vi "Transmission.vi"() -> ()   [LabVIEW 2016, in "beamline sections.lvlib" / "transmission.lvlib"]
uses:
  Transmission/transmission.lvlib
  save load/saveloadprev.ctl
  controls/Faraday cup states.ctl
  <vilib>/Instr/_visa.llb/VISA Open Access Mode.ctl
  low energy end/Low energy end/Low energy end llb.lvlib
  High energy end/High energy llb.lvlib
  save load/SaveLoad.lvlib
panel:
  in  "Tab Control":T1(tab)
  in  "ExB Electric":dbl(slide) min=0.0 max=200.0 scale=0.0..60.0
  out "Trans Steerer Y Read":dbl format="%#.3g"
  out "Trans Steerer X Read":dbl format="%#.3g"
  in  "Transmission Y steerer":dbl(slide) min=-10.0 max=10.0 scale=-10.0..10.0
  in  "Transmission Quad A":dbl(slide) min=0.0 max=200.0 scale=0.0..120.0
  out "Switch magnet":bool=TRUE
  in  "Transmission X steerer":dbl(slide) min=-10.0 max=10.0 scale=-10.0..10.0
  out "Transmission Steerer":bool
  out "Transmission quad Range":bool
  in  "Transmission Quad B":dbl(slide) min=0.0 max=200.0 scale=0.0..120.0
  in  "stop":bool
  out "ExB":bool
  out "ExB Voltage Read-":dbl format="%#.3g"
  in  "ExB Magnet":dbl(slide) scale=0.0..10.0
  out "ExB Voltage Read +":dbl format="%#.3g"
  in  "Switch magnet set":dbl(slide) min=0.0 max=1.6 scale=0.0..1.0
  out "Switch magnet readback":dbl(graph)
  out "Quad A I read":string
  out "Quad A V read":string
  out "Quad B I read":string
  out "Quad B V read":string
  in  "Preview-Save-Load":T2
  out "ExB Magnet read":dbl
  out "R30 Switch magnet FC status":T3
  out "Switch Mag PS output setting":dbl
  in  "Trans temp file":path=path "D:/Main Tune Parameters/Temp Configs/Transmission.txt"
  in  "Quad A - VISA GPIB Resource":refnum<visa-resource-name>="GPIB2::8::INSTR"
  in  "Quad B - VISA GPIB Resource":refnum<visa-resource-name>="GPIB2::12::INSTR"
  out "ExB +READ I":dbl
  out "ExB - I":dbl
  out "Trans steer +X I":dbl
  out "Trans steer -X  I":dbl
  out "Trans steer +Y I":dbl
  out "Trans steer -Y I":dbl
  out "Trans steer +X":dbl
  out "Trans steer -X":dbl
  out "Trans steer +X Set":dbl
  out "Trans steer -X Set":dbl
  out "Trans steer +Y":dbl
  out "Trans steer -Y":dbl
  out "Trans steer +Y Set":dbl
  out "Trans steer -Y Set":dbl
  out "Quad B error":errorcluster
  out "Quad A error":errorcluster
  out "SaveLoad error":errorcluster
  out "SV error - event loop":errorcluster
  out "SV error - while loop":errorcluster
  out "Trans-RT Error":errorcluster
  out "Trans-FPGA Error":errorcluster
  # "Transmission"
  # "Quad A initially set to GPIB2::8\nQuad B initially set to GPIB2::12"
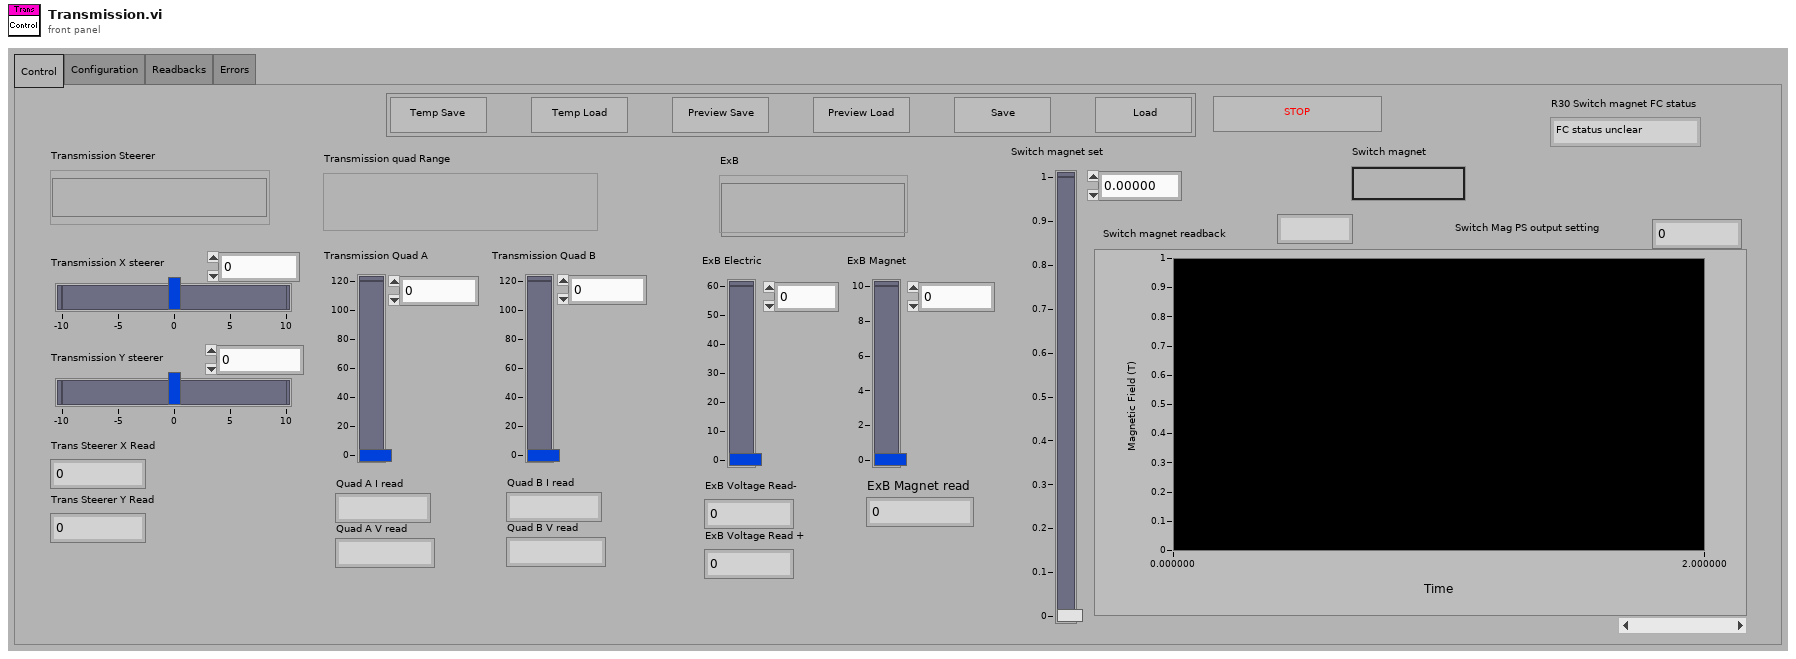
[diagram p1: front panel]
types:
  T1 = enum32{"Control", "Configuration", "Readbacks", "Errors"}
  T2 = typedef "saveloadprev.ctl" = cluster{"Temp Save":bool, "Temp Load":bool, "Save":bool, "Load":bool, "Preview Save":bool, "Preview Load":bool}
  T3 = typedef "Faraday cup states.ctl" = enum16{"FC status unclear", "FC in", "FC out"}
  T4 = typedef "VISA Open Access Mode.ctl" = u32
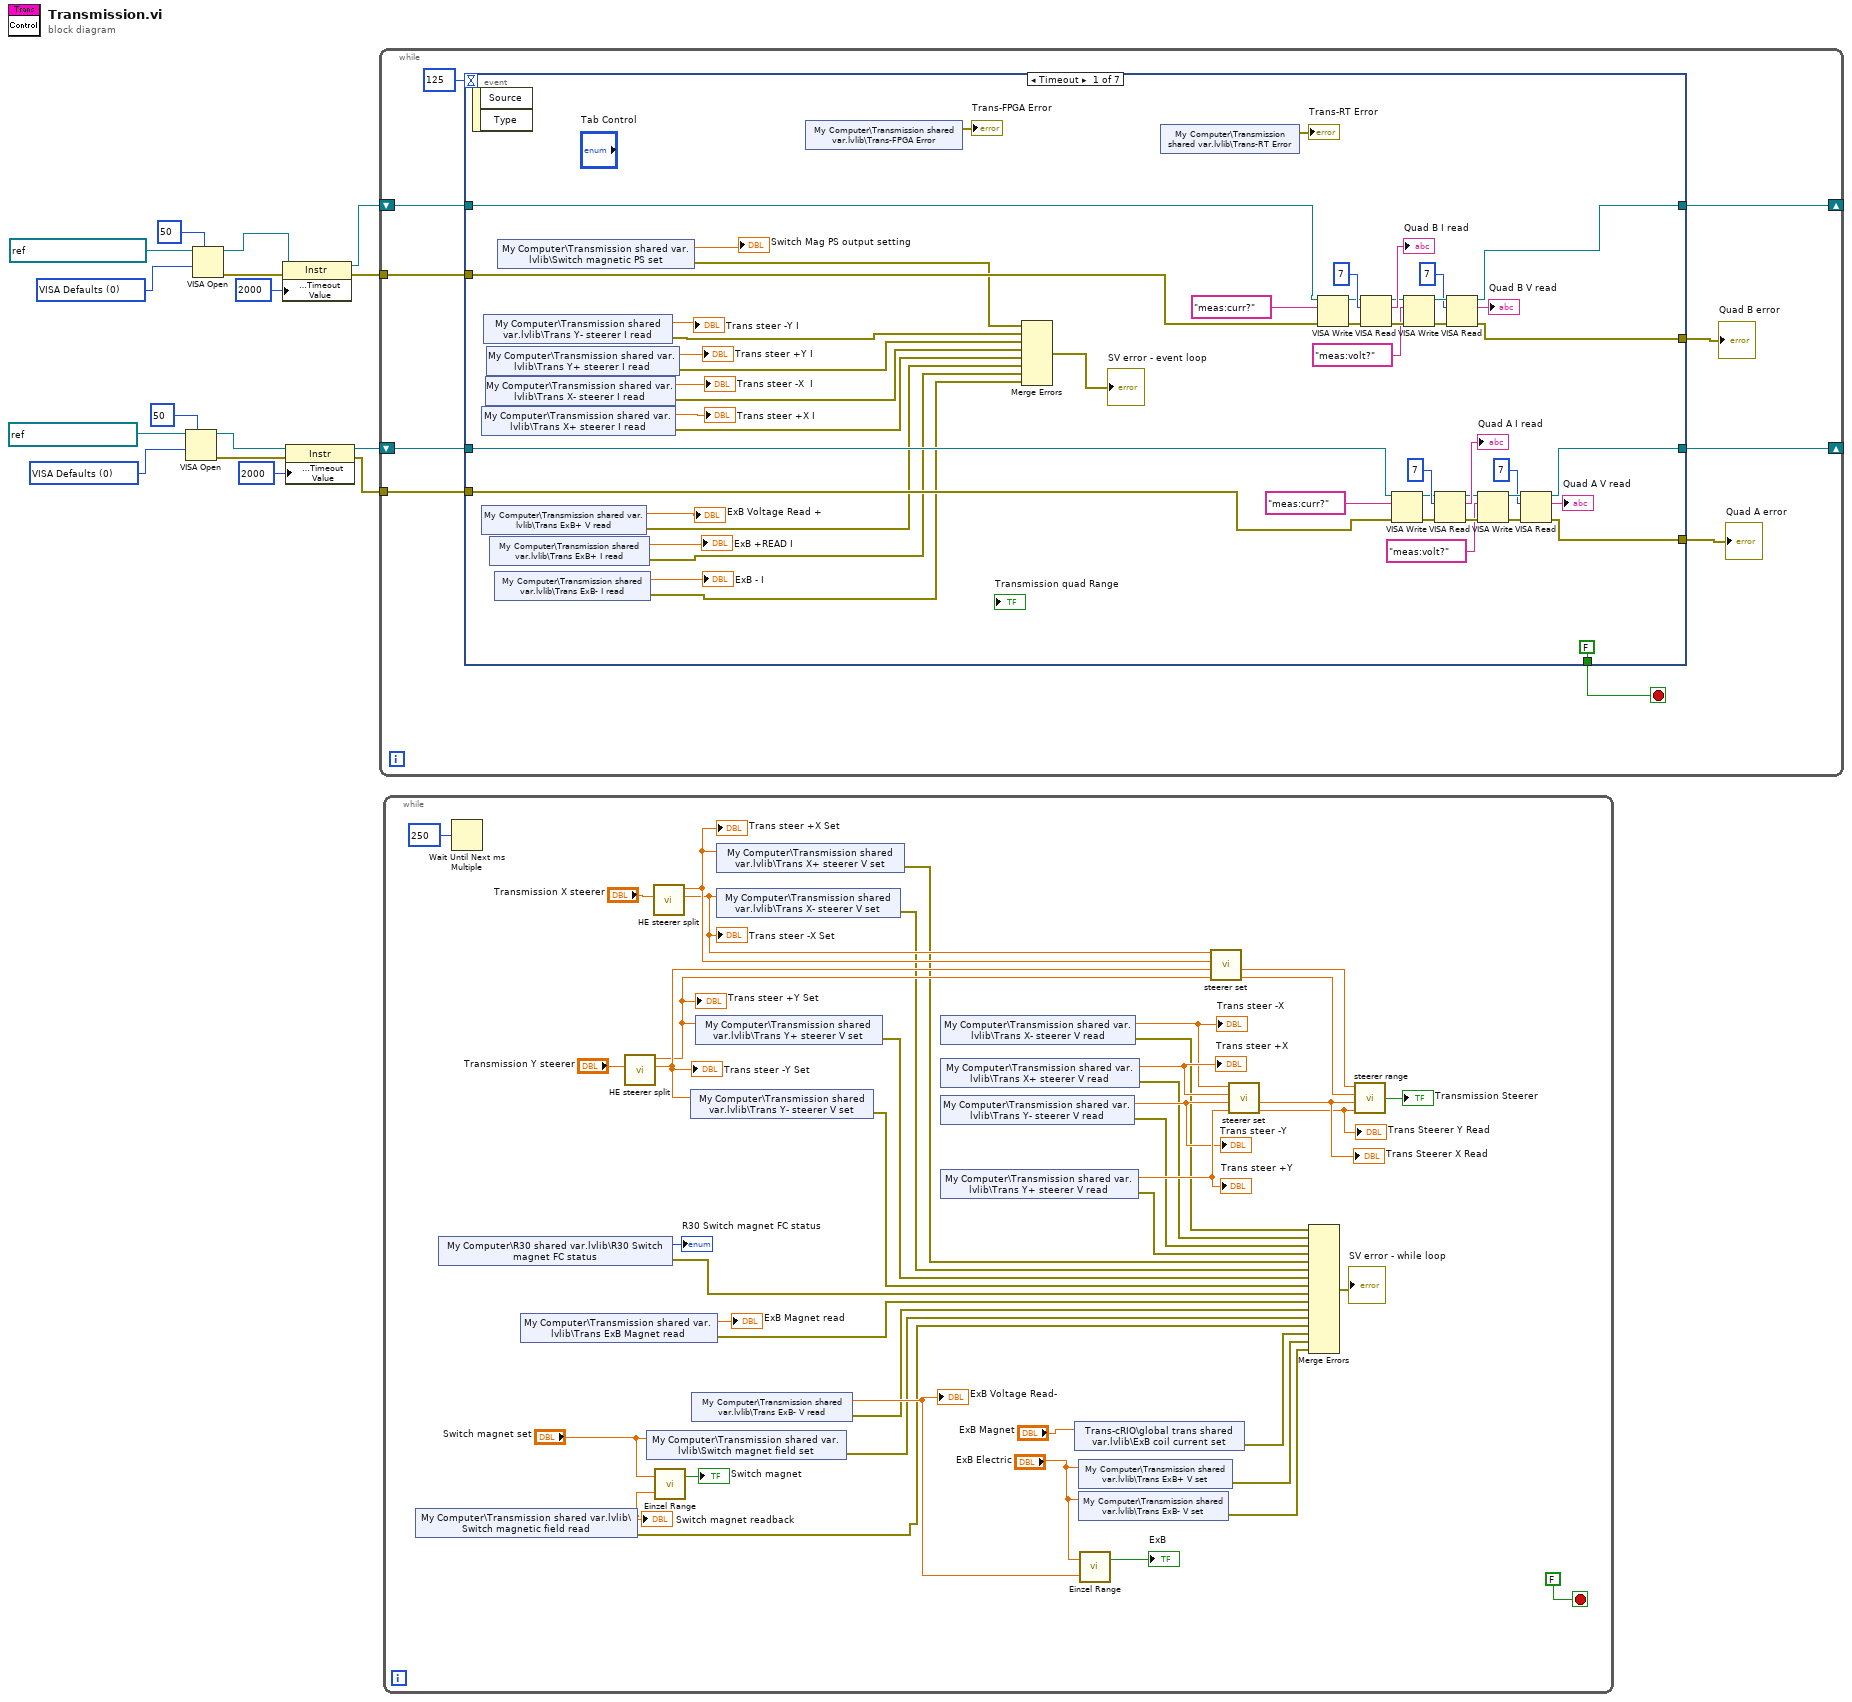
[diagram p0: block diagram]
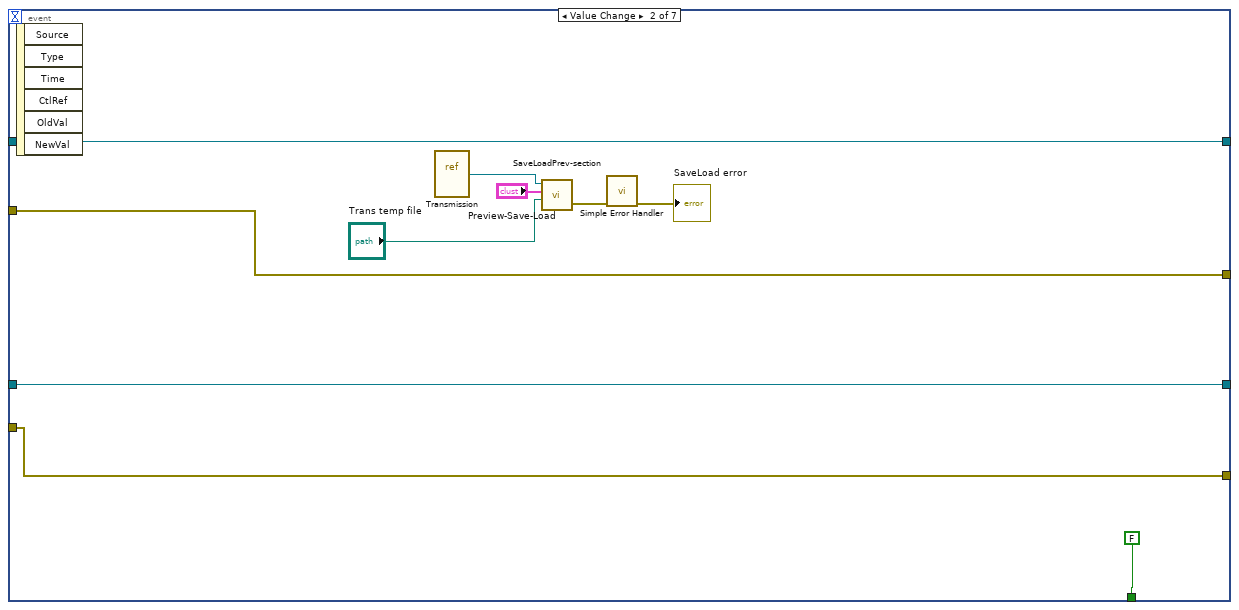
[diagram p2: hidden frame]
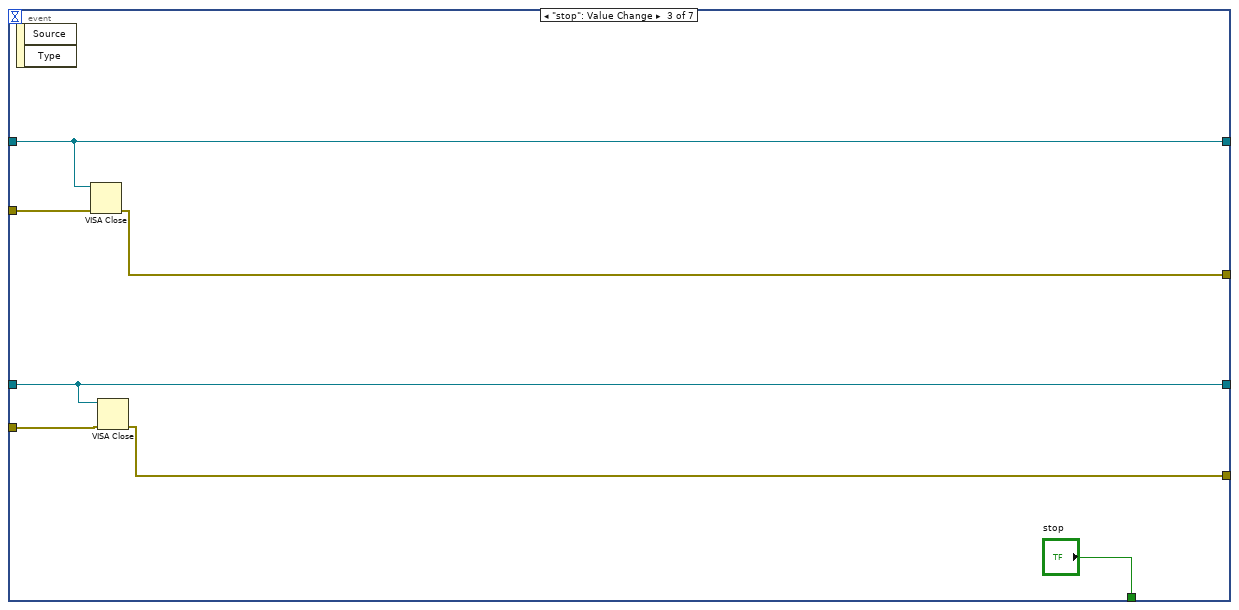
[diagram p3: hidden frame]
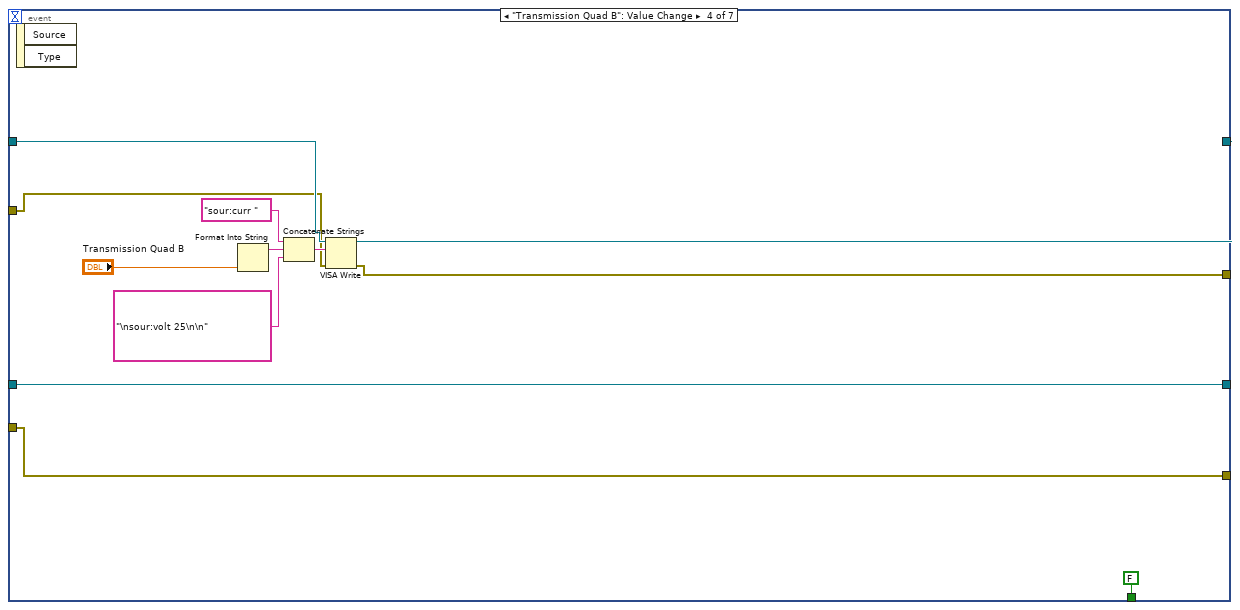
[diagram p4: hidden frame]
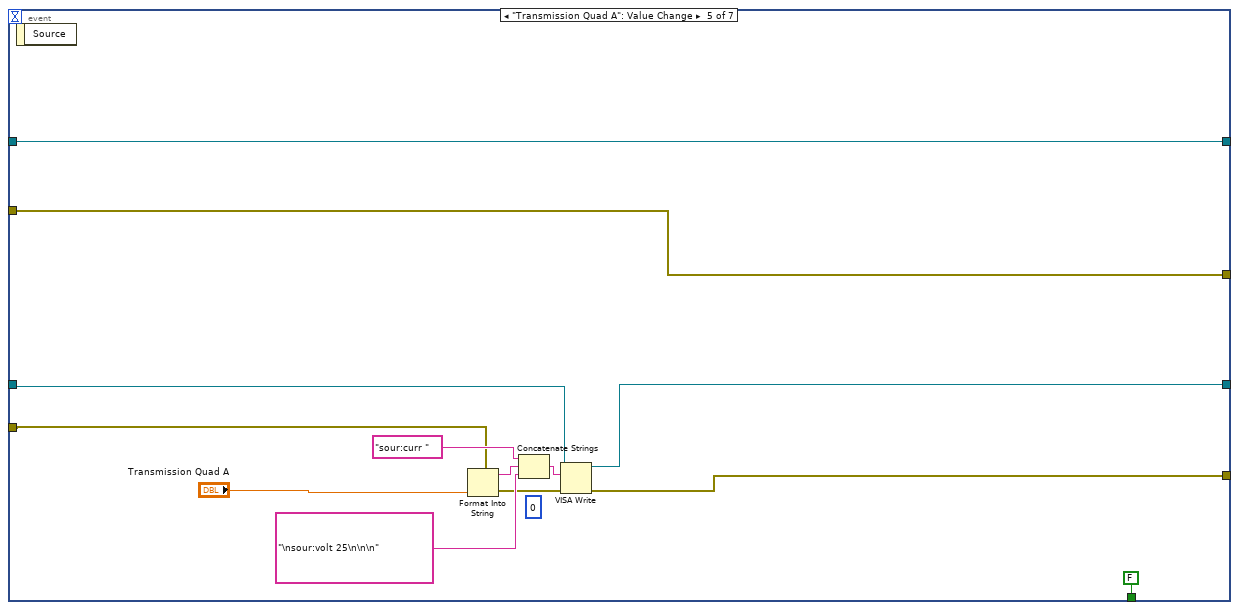
[diagram p5: hidden frame]
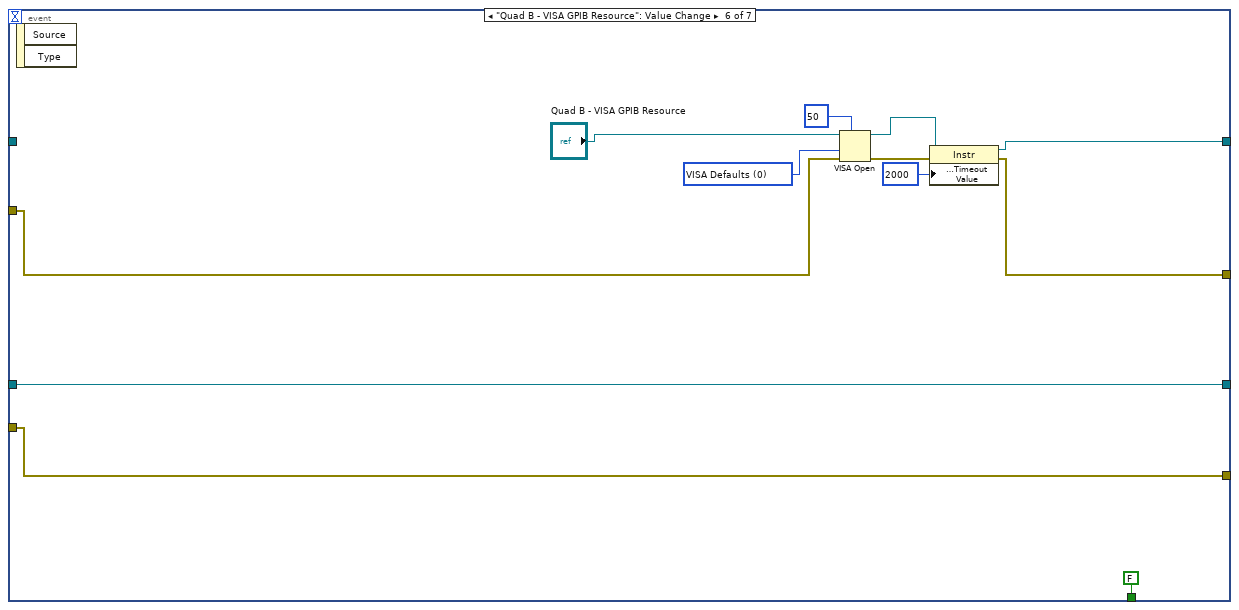
[diagram p6: hidden frame]
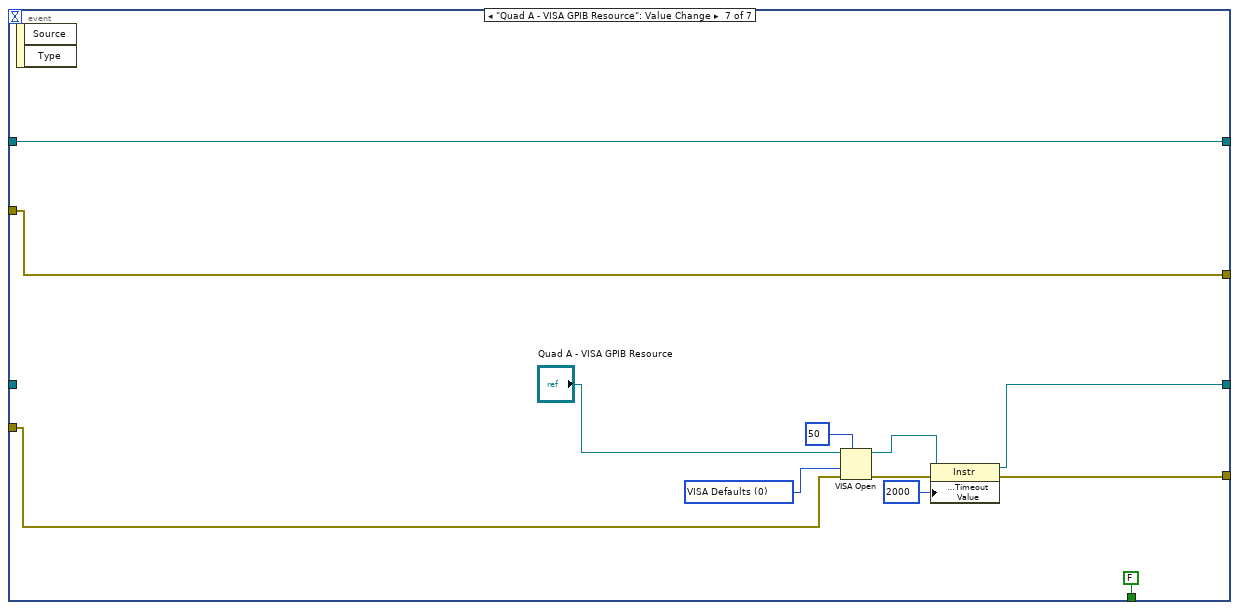
[diagram p7: hidden frame]
diagram:
  w8 = T4 0 items=["VISA Defaults"=0, "Exclusive Lock"=1, "Load Configured Settings"=4] ("Access Mode")
  w16 = T4 0 items=["VISA Defaults"=0, "Exclusive Lock"=1, "Load Configured Settings"=4] ("Access Mode")
  n1 = VISA Open(timeout (0)=u32 50 ("VISA Open timeout (0)"), access mode=w16, VISA resource name=refnum<visa-resource-name> "GPIB2::8::INSTR" ("Quad A - VISA GPIB Resource 2")) -> (VISA resource name=w13:refnum<visa-resource-name>, error out=w12:errorcluster)  [unwired: 2 in]
  n2 = VISA Open(timeout (0)=u32 50 ("VISA Open timeout (0)"), access mode=w8, VISA resource name=refnum<visa-resource-name> "GPIB2::12::INSTR" ("Quad B - VISA GPIB Resource 2")) -> (VISA resource name=w10:refnum<visa-resource-name>, error out=w11:errorcluster)  [unwired: 2 in]
  n3 = property class="Instr"(reference=w10, error in=w11, "General Settings:Timeout Value"=u32 2000) -> (reference out=w6:refnum<visa-resource-name>, error out=w5:errorcluster)
  n4 = property class="Instr"(reference=w13, error in=w12, "General Settings:Timeout Value"=u32 2000) -> (reference out=w4:refnum<visa-resource-name>, error out=w3:errorcluster)
  n5 = while {
    tunnel: w5 -> [w24]
    tunnel: w3 -> [w22]
    shift-right: [w21] -> _
    shift-left: w6 -> [w25]
    shift-right: [w20] -> _
    shift-left: w4 -> [w23]
    stop <- w26 stop-if-true
    n6 = event shown="[0] Timeout" {
      selector: _ -> [_ _ _ _ _ _ _]
      dyn-events: _ -> [_ _ _ _ _ _ _]
      timeout: 125 -> [_ _ _ _ _ _ _]
      tunnel: [FALSE ("stop") FALSE ("stop") "stop" FALSE ("stop") FALSE ("stop") FALSE ("stop") FALSE ("stop")] -> w26
      tunnel: w25 -> [w40 w87 w92 w102 w109 _ w142]
      tunnel: w24 -> [w41 w86 w94 w101 w110 w121 w143]
      tunnel: w23 -> [w57 w85 w91 w100 w114 w130 _]
      tunnel: w22 -> [w56 w84 w93 w99 w113 w131 w132]
      tunnel: [w43 w87 w92 w98 w109 w122 w142] -> w21
      tunnel: [w58 w85 w91 w100 w111 w130 w134] -> w20
      tunnel: [w42 w86 w90 w97 w110 w120 w143] -> w19
      tunnel: [w59 w84 w89 w99 w112 w131 w133] -> w18
      event Timeout {
        n7 = event-data() -> ()  [unwired: 1 in, 2 out]
        n8 = shared-variable "My Computer\\Transmission shared var.lvlib\\Trans X+ steerer I read"() -> (→"Trans steer +X I":dbl, error out=w33:errorcluster)  [unwired: 1 in]
        n9 = shared-variable "My Computer\\Transmission shared var.lvlib\\Trans ExB+ V read"() -> (→"ExB Voltage Read +":dbl, error out=w32:errorcluster)  [unwired: 1 in]
        n10 = shared-variable "My Computer\\Transmission shared var.lvlib\\Trans Y- steerer I read"() -> (→"Trans steer -Y I":dbl, error out=w36:errorcluster)  [unwired: 1 in]
        n11 = shared-variable "My Computer\\Transmission shared var.lvlib\\Trans X- steerer I read"() -> (→"Trans steer -X  I":dbl, error out=w34:errorcluster)  [unwired: 1 in]
        n12 = shared-variable "My Computer\\Transmission shared var.lvlib\\Trans Y+ steerer I read"() -> (→"Trans steer +Y I":dbl, error out=w35:errorcluster)  [unwired: 1 in]
        n13 = shared-variable "My Computer\\Transmission shared var.lvlib\\Trans ExB+ I read"() -> (→"ExB +READ I":dbl, error out=w31:errorcluster)  [unwired: 1 in]
        n14 = shared-variable "My Computer\\Transmission shared var.lvlib\\Trans ExB- I read"() -> (→"ExB - I":dbl, error out=w30:errorcluster)  [unwired: 1 in]
        n15 = shared-variable "My Computer\\Transmission shared var.lvlib\\Switch magnetic PS set"() -> (→"Switch Mag PS output setting":dbl, error out=w37:errorcluster)  [unwired: 1 in]
        n16 = shared-variable "My Computer\\Transmission shared var.lvlib\\Trans-FPGA Error"() -> (→"Trans-FPGA Error":errorcluster)  [unwired: 1 in, 1 out]
        n17 = Merge Errors(w37, w36, w35, w34, w33, w32, w31, w30) -> (→"SV error - event loop":errorcluster)
        n18 = shared-variable "My Computer\\Transmission shared var.lvlib\\Trans-RT Error"() -> (→"Trans-RT Error":errorcluster)  [unwired: 1 in, 1 out]
        n19 = VISA Write(VISA resource name=w40, write buffer="meas:curr?", error in (no error)=w41) -> (VISA resource name out=w52:refnum<visa-resource-name>, error out=w53:errorcluster)  [unwired: 1 out]
        n20 = VISA Read(VISA resource name=w52, byte count=u32 7, error in (no error)=w53) -> (VISA resource name out=w48:refnum<visa-resource-name>, read buffer=→"Quad B I read":string, error out=w47:errorcluster)  [unwired: 1 out]
        n21 = VISA Write(VISA resource name=w57, write buffer="meas:curr?", error in (no error)=w56) -> (VISA resource name out=w68:refnum<visa-resource-name>, error out=w69:errorcluster)  [unwired: 1 out]
        n22 = VISA Write(VISA resource name=w48, write buffer="meas:volt?", error in (no error)=w47) -> (VISA resource name out=w50:refnum<visa-resource-name>, error out=w45:errorcluster)  [unwired: 1 out]
        n23 = VISA Read(VISA resource name=w68, byte count=u32 7, error in (no error)=w69) -> (VISA resource name out=w64:refnum<visa-resource-name>, read buffer=→"Quad A I read":string, error out=w63:errorcluster)  [unwired: 1 out]
        n24 = VISA Read(VISA resource name=w50, byte count=u32 7, error in (no error)=w45) -> (VISA resource name out=w43:refnum<visa-resource-name>, read buffer=→"Quad B V read":string, error out=w42:errorcluster)  [unwired: 1 out]
        n25 = VISA Write(VISA resource name=w64, write buffer="meas:volt?", error in (no error)=w63) -> (VISA resource name out=w66:refnum<visa-resource-name>, error out=w61:errorcluster)  [unwired: 1 out]
        n26 = VISA Read(VISA resource name=w66, byte count=u32 7, error in (no error)=w61) -> (VISA resource name out=w58:refnum<visa-resource-name>, read buffer=→"Quad A V read":string, error out=w59:errorcluster)  [unwired: 1 out]
      }
      event Value Change {
        n27 = event-data() -> ()  [unwired: 1 in, 6 out]
        n28 = vi-ref "Transmission.vi"() -> (w82:refnum<vi>)
        n29 = call "SaveLoadPrev-section.vi"("file path (use dialog)"="Trans temp file", "Cluster 2"="Preview-Save-Load", "VI Refnum"=w82) -> ("error out"=w80:errorcluster)  [unwired: 2 in]
        n30 = call <vilib>:"Simple Error Handler.vi"("error in (no error)"=w80) -> ("error out"=→"SaveLoad error":errorcluster)  [unwired: 4 in, 4 out]
      }
      event "stop": Value Change {
        n31 = event-data() -> ()  [unwired: 1 in, 2 out]
        n32 = VISA Close(VISA resource name=w92, error in (no error)=w94) -> (error out=w90:errorcluster)
        n33 = VISA Close(VISA resource name=w91, error in (no error)=w93) -> (error out=w89:errorcluster)
      }
      event "Transmission Quad B": Value Change {
        n34 = event-data() -> ()  [unwired: 1 in, 2 out]
        n35 = Format Into String("Transmission Quad B") -> (resulting string=w105:string)  [unwired: 3 in, 1 out]
        n36 = Concatenate Strings("sour:curr " ("string"), w105, "\nsour:volt 25\n\n" ("write buffer")) -> (w104:string)
        n37 = VISA Write(VISA resource name=w102, write buffer=w104, error in (no error)=w101) -> (VISA resource name out=w98:refnum<visa-resource-name>, error out=w97:errorcluster)  [unwired: 1 out]
      }
      event "Transmission Quad A": Value Change {
        (unwired) i16 0 ("mode (0)")
        n38 = event-data() -> ()  [unwired: 1 in, 1 out]
        n39 = Format Into String("Transmission Quad A") -> (resulting string=w116:string)  [unwired: 3 in, 1 out]
        n40 = Concatenate Strings("sour:curr " ("string"), w116, "\nsour:volt 25\n\n\n" ("write buffer")) -> (w118:string)
        n41 = VISA Write(VISA resource name=w114, write buffer=w118, error in (no error)=w113) -> (VISA resource name out=w111:refnum<visa-resource-name>, error out=w112:errorcluster)  [unwired: 1 out]
      }
      event "Quad B - VISA GPIB Resource": Value Change {
        w125 = T4 0 items=["VISA Defaults"=0, "Exclusive Lock"=1, "Load Configured Settings"=4] ("Access Mode")
        n42 = event-data() -> ()  [unwired: 1 in, 2 out]
        n43 = VISA Open(timeout (0)=u32 50 ("VISA Open timeout (0)"), access mode=w125, error in (no error)=w121, VISA resource name="Quad B - VISA GPIB Resource") -> (VISA resource name=w127:refnum<visa-resource-name>, error out=w128:errorcluster)  [unwired: 1 in]
        n44 = property class="Instr"(reference=w127, error in=w128, "General Settings:Timeout Value"=u32 2000) -> (reference out=w122:refnum<visa-resource-name>, error out=w120:errorcluster)
      }
      event "Quad A - VISA GPIB Resource": Value Change {
        w137 = T4 0 items=["VISA Defaults"=0, "Exclusive Lock"=1, "Load Configured Settings"=4] ("Access Mode")
        n45 = event-data() -> ()  [unwired: 1 in, 2 out]
        n46 = VISA Open(timeout (0)=u32 50 ("VISA Open timeout (0)"), access mode=w137, error in (no error)=w132, VISA resource name="Quad A - VISA GPIB Resource") -> (VISA resource name=w139:refnum<visa-resource-name>, error out=w140:errorcluster)  [unwired: 1 in]
        n47 = property class="Instr"(reference=w139, error in=w140, "General Settings:Timeout Value"=u32 2000) -> (reference out=w134:refnum<visa-resource-name>, error out=w133:errorcluster)
      }
    }
    "Quad B error" <- w19
    "Quad A error" <- w18
  }
  n48 = while {
    stop <- FALSE stop-if-true
    n49 = shared-variable "My Computer\\Transmission shared var.lvlib\\Switch magnetic field read"() -> (w167:dbl, error out=w154:errorcluster)  [unwired: 1 in]
    "Switch magnet readback" <- w167
    n50 = shared-variable "My Computer\\R30 shared var.lvlib\\R30 Switch magnet FC status"() -> (→"R30 Switch magnet FC status":T3, error out=w155:errorcluster)  [unwired: 1 in]
    n51 = Wait Until Next ms Multiple(millisecond multiple=u32 250) -> ()  [unwired: 1 out]
    n52 = shared-variable "My Computer\\Transmission shared var.lvlib\\Trans ExB Magnet read"() -> (→"ExB Magnet read":dbl, error out=w147:errorcluster)  [unwired: 1 in]
    n53 = call "HE steerer split.vi"("Steerer in"="Transmission Y steerer") -> ("Steerer +"=w170:dbl, "Steerer -"=w171:dbl)  [unwired: 7 in]
    "Trans steer +Y Set" <- w170
    "Trans steer -Y Set" <- w171
    n54 = shared-variable "My Computer\\Transmission shared var.lvlib\\Switch magnet field set"("Switch magnet set") -> (error out=w153:errorcluster)  [unwired: 1 in]
    n55 = call "HE steerer split.vi"("Steerer in"="Transmission X steerer") -> ("Steerer +"=w173:dbl, "Steerer -"=w172:dbl)  [unwired: 7 in]
    "Trans steer +X Set" <- w173
    "Trans steer -X Set" <- w172
    n56 = call "Einzel Range.vi"("Inj image Readback"=w167, "Inj image Einzel Set"="Switch magnet set") -> ("Einzel  Range"=→"Switch magnet":bool)  [unwired: 1 out]
    n57 = shared-variable "My Computer\\Transmission shared var.lvlib\\Trans Y- steerer V set"(w171) -> (error out=w156:errorcluster)  [unwired: 1 in]
    n58 = shared-variable "My Computer\\Transmission shared var.lvlib\\Trans ExB- V read"() -> (w166:dbl, error out=w152:errorcluster)  [unwired: 1 in]
    "ExB Voltage Read-" <- w166
    n59 = shared-variable "My Computer\\Transmission shared var.lvlib\\Trans Y+ steerer V set"(w170) -> (error out=w157:errorcluster)  [unwired: 1 in]
    n60 = shared-variable "My Computer\\Transmission shared var.lvlib\\Trans X+ steerer V set"(w173) -> (error out=w159:errorcluster)  [unwired: 1 in]
    n61 = shared-variable "My Computer\\Transmission shared var.lvlib\\Trans X- steerer V set"(w172) -> (error out=w158:errorcluster)  [unwired: 1 in]
    n62 = shared-variable "My Computer\\Transmission shared var.lvlib\\Trans X- steerer V read"() -> (w179:dbl, error out=w163:errorcluster)  [unwired: 1 in]
    "Trans steer -X" <- w179
    n63 = shared-variable "My Computer\\Transmission shared var.lvlib\\Trans X+ steerer V read"() -> (w180:dbl, error out=w162:errorcluster)  [unwired: 1 in]
    "Trans steer +X" <- w180
    n64 = shared-variable "My Computer\\Transmission shared var.lvlib\\Trans Y- steerer V read"() -> (w177:dbl, error out=w161:errorcluster)  [unwired: 1 in]
    "Trans steer -Y" <- w177
    n65 = shared-variable "My Computer\\Transmission shared var.lvlib\\Trans Y+ steerer V read"() -> (w178:dbl, error out=w160:errorcluster)  [unwired: 1 in]
    "Trans steer +Y" <- w178
    n66 = shared-variable "Trans-cRIO\\global trans shared var.lvlib\\ExB coil current set"("ExB Magnet") -> (error out=w144:errorcluster)  [unwired: 1 in]
    n67 = shared-variable "My Computer\\Transmission shared var.lvlib\\Trans ExB+ V set"("ExB Electric") -> (error out=w151:errorcluster)  [unwired: 1 in]
    n68 = shared-variable "My Computer\\Transmission shared var.lvlib\\Trans ExB- V set"("ExB Electric") -> (error out=w150:errorcluster)  [unwired: 1 in]
    n69 = call "Einzel Range.vi"("Inj image Readback"=w166, "Inj image Einzel Set"="ExB Electric") -> ("Einzel  Range"=→"ExB":bool)  [unwired: 1 out]
    n70 = call "steerer set.vi"("Injector image X  -"=w172, "Injector image X +"=w173, "Injector image Y  -"=w171, "Injector image Y +"=w170) -> ("Steerer X"=w184:dbl, "Steerer Y"=w183:dbl)  [unwired: 4 out]
    n71 = call "steerer set.vi"("Injector image X  -"=w179, "Injector image X +"=w180, "Injector image Y  -"=w177, "Injector image Y +"=w178) -> ("Steerer X"=w176:dbl, "Steerer Y"=w175:dbl)  [unwired: 4 out]
    "Trans Steerer X Read" <- w176
    "Trans Steerer Y Read" <- w175
    n72 = Merge Errors(w163, w162, w161, w160, w159, w158, w157, w156, w155, w147, w152, w153, w154, w144, w151, w150) -> (→"SV error - while loop":errorcluster)
    n73 = call "steerer range.vi"("Steerer Y Voltage"=w175, "Steerer X Voltage"=w176, "Steerer Set Y"=w183, "Steerer X Set"=w184) -> ("Steerer within range"=→"Transmission Steerer":bool)  [unwired: 3 out]
  }
